vi "Configure Modulation (Burst).vi"(0 "VISA resource name":refnum<visa-resource-name>, 1 "Burst Phase (0 deg)":i32 min=-360 max=360, 2 "Burst Count (1)":i32=1, 3 "Burst Period (1 s)":dbl=1.0 min=0.002 max=1000000.0 format="%.6f", 5 "Enable Burst Modulation (T: Enable)":bool=TRUE, 7 "Burst Modulation Mode (0: Triggered)":u16(ring) items=["Triggered", "Gated"], 11 "error in (no error)":errorcluster) -> (4 "VISA resource name out":refnum<visa-resource-name>, 15 "error out":errorcluster)   [LabVIEW 2018, in "AWG.lvlib" / "Agilent 33XXX Series.lvlib"]
doc: "Allows and configures burst modulation. Configures the function generator to output a waveform with specified number of cycles, called burst. The carrier waveform shape and parameters are set by Configure Standard Waveform. When -1 is set to 'burst count' it will enable continuous burst mode.\n\nNote:\n(1) Before using this mode, all other modes must be turned off.\n(2) This VI is not valid in 33210."
uses:
  Agilent 33XXX Series.lvlib
panel:
  # "Triggered BM Settings"
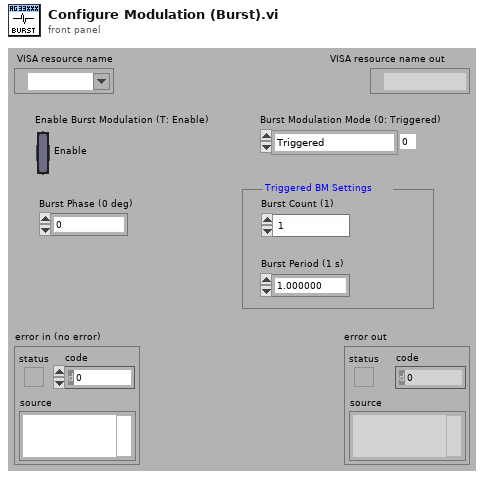
[diagram p1: front panel]
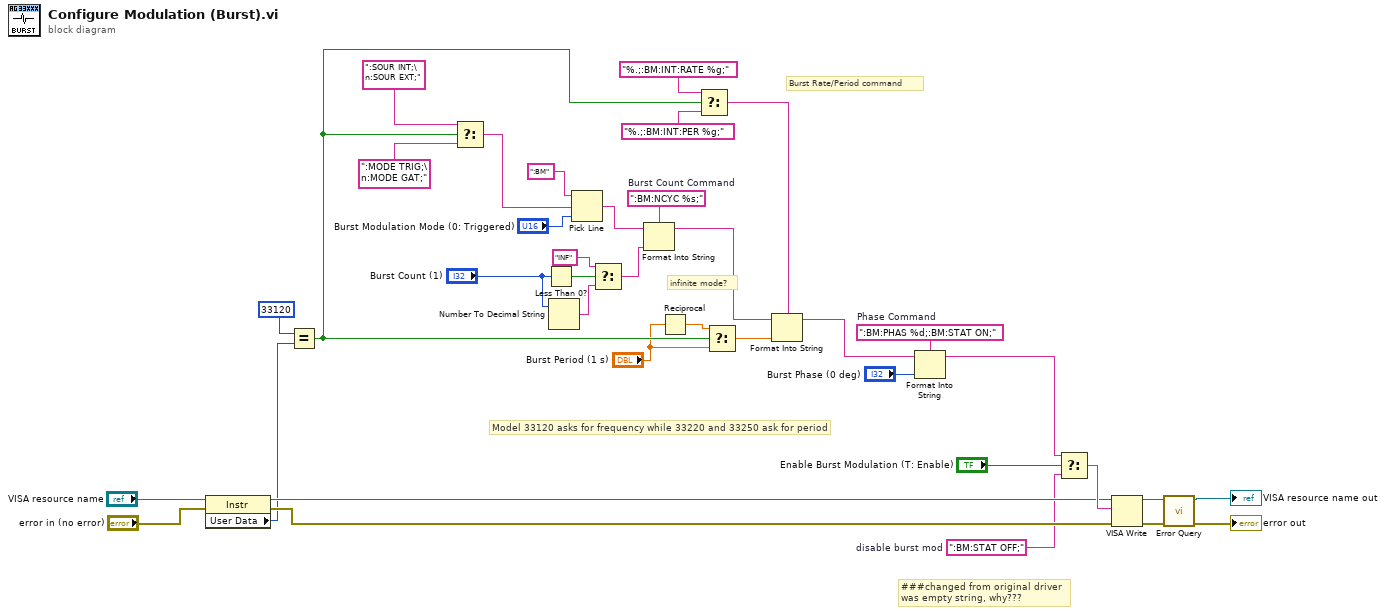
[diagram p0: block diagram]
diagram:
  w1 = ":BM:STAT OFF;"  # disable burst mod
  w34 = ":BM:PHAS %d;:BM:STAT ON;"  # Phase Command
  w35 = ":BM:NCYC %s;"  # Burst Count Command
  # "###changed from original driver\nwas empty string, why???"
  # "infinite mode?"
  # "Model 33120 asks for frequency while 33220 and 33250 ask for period"
  # "Burst Rate/Period command"
  n1 = property class="Instr"(reference="VISA resource name", error in="error in (no error)") -> (reference out=w30:refnum<visa-resource-name>, error out=w29:errorcluster, "User Data"=w28:u32)
  n2 = Equal?(x=u32 33120, y=w28) -> (x = y?=w19:bool)
  n3 = Select(t=":SOUR INT;\n:SOUR EXT;" ("Source Command"), s=w19, f=":MODE TRIG;\n:MODE GAT;") -> (s? t:f=w24:string)
  n4 = Less Than 0?(x="Burst Count (1)") -> (x < 0?=w5:bool)
  n5 = Number To Decimal String(number="Burst Count (1)") -> (decimal integer string=w3:string)  [unwired: 1 in]
  n6 = Pick Line(string ("")=":BM", multi-line string=w24, line index="Burst Modulation Mode (0: Triggered)") -> (output string=w23:string)
  n7 = Select(t="INF", s=w5, f=w3) -> (s? t:f=w6:string)
  n8 = Format Into String(format string=w35, initial string=w23, w6) -> (resulting string=w15:string)  [unwired: 1 in, 1 out]
  n9 = Reciprocal(x="Burst Period (1 s)") -> (1/x=w18:dbl)
  n10 = Select(t="%.;:BM:INT:RATE %g;" ("Rate Command"), s=w19, f="%.;:BM:INT:PER %g;") -> (s? t:f=w20:string)
  n11 = Select(t=w18, s=w19, f="Burst Period (1 s)") -> (s? t:f=w16:dbl)
  n12 = Format Into String(format string=w20, initial string=w15, w16) -> (resulting string=w14:string)  [unwired: 1 in, 1 out]
  n13 = Format Into String(format string=w34, initial string=w14, "Burst Phase (0 deg)") -> (resulting string=w13:string)  [unwired: 1 in, 1 out]
  n14 = Select(t=w13, s="Enable Burst Modulation (T: Enable)", f=w1) -> (s? t:f=w32:string)
  n15 = VISA Write(VISA resource name=w30, write buffer=w32, error in (no error)=w29) -> (VISA resource name out=w37:refnum<visa-resource-name>, error out=w36:errorcluster)  [unwired: 1 out]
  n16 = call "Error Query.vi"("error in (no error)"=w36, "VISA resource name"=w37) -> ("error out"=→"error out":errorcluster, "VISA resource name out"=→"VISA resource name out":refnum<visa-resource-name>)  [unwired: 6 in, 2 out]
